vi "XML Read.vi"(8 "error in":errorcluster, 11 "XML File Path In":path) -> (0 "error out":errorcluster, 3 "FOFB Parameters":T1)   [LabVIEW 2011, in "XML VIs.lvlib"]
doc: "Reads an XML file coitaning the FOFB configuration parameters and builds a raw configuration cluster (FOFB Parameters)."
uses:
  XML VIs.lvlib
  Types Definitions/Type FOFB Parameters.ctl
  Types Definitions/Type Network Configuration.ctl
  Types Definitions/Type FA Configuration.ctl
  Types Definitions/Type Response Matrix Measurement Configuration.ctl
  Types Definitions/Type Correction Algorithm Configuration.ctl
  Types Definitions/Type Acquisition Network Configuration.ctl
  Types Definitions/Type Actuation Network Configuration.ctl
  Third Party/GXML/_subVIis/GXML SearchParser/gxml_SearchParser.vi
  Third Party/GXML/GXML.lvlib
  Type Definitions.lvlib
  Controller VIs.lvlib
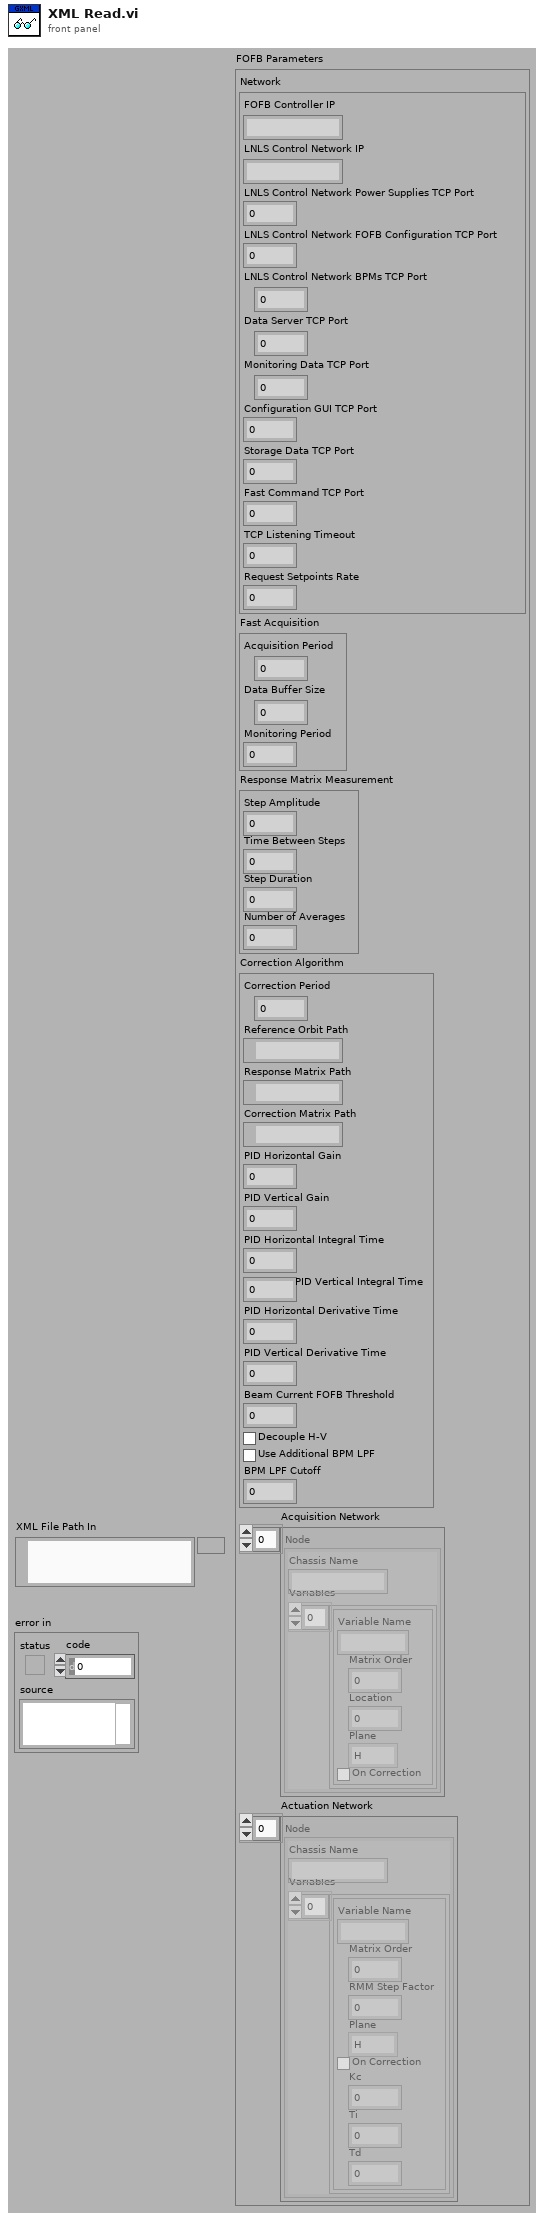
[diagram p1: front panel]
types:
  T1 = typedef "Type Definitions.lvlib/Type FOFB Parameters.ctl" = cluster{"Network":T2, "Fast Acquisition":T3, "Response Matrix Measurement":T4, "Correction Algorithm":T5, "Acquisition Network":T6, "Actuation Network":T7}
  T2 = typedef "Type Definitions.lvlib/Type Network Configuration.ctl" = cluster{"FOFB Controller IP":string, "LNLS Control Network IP":string, "LNLS Control Network Power Supplies TCP Port":u16, "LNLS Control Network FOFB Configuration TCP Port":u16, "LNLS Control Network BPMs TCP Port":u16, "Data Server TCP Port":u16, "Monitoring Data TCP Port":u16, "Configuration GUI TCP Port":u16, "Storage Data TCP Port":u16, "Fast Command TCP Port":u16, "TCP Listening Timeout":i32, "Request Setpoints Rate":u16}
  T3 = typedef "Type Definitions.lvlib/Type FA Configuration.ctl" = cluster{"Acquisition Period":u32, "Data Buffer Size":u32, "Monitoring Period":u32}
  T4 = typedef "Type Definitions.lvlib/Type Response Matrix Measurement Configuration.ctl" = cluster{"Step Amplitude":dbl, "Time Between Steps":u32, "Step Duration":u32, "Number of Averages":u32}
  T5 = typedef "Type Definitions.lvlib/Type Correction Algorithm Configuration.ctl" = cluster{"Correction Period":u32, "Reference Orbit Path":path, "Response Matrix Path":path, "Correction Matrix Path":path, "PID Horizontal Gain":dbl, "PID Vertical Gain":dbl, "PID Horizontal Integral Time":dbl, "PID Vertical Integral Time":dbl, "PID Horizontal Derivative Time":dbl, "PID Vertical Derivative Time":dbl, "Beam Current FOFB Threshold":dbl, "Decouple H-V":bool, "Use Additional BPM LPF":bool, "BPM LPF Cutoff":dbl}
  T6 = typedef "Type Definitions.lvlib/Type Acquisition Network Configuration.ctl" = cluster{"Chassis Name":string, "Variables":cluster{"Variable Name":string, "Matrix Order":u32, "Location":dbl, "Plane":enum8{"H", "V"}, "On Correction":bool}[]}[]
  T7 = typedef "Type Definitions.lvlib/Type Actuation Network Configuration.ctl" = cluster{"Chassis Name":string, "Variables":cluster{"Variable Name":string, "Matrix Order":u32, "RMM Step Factor":dbl, "Plane":enum8{"H", "V"}, "On Correction":bool, "Kc":dbl, "Ti":dbl, "Td":dbl}[]}[]
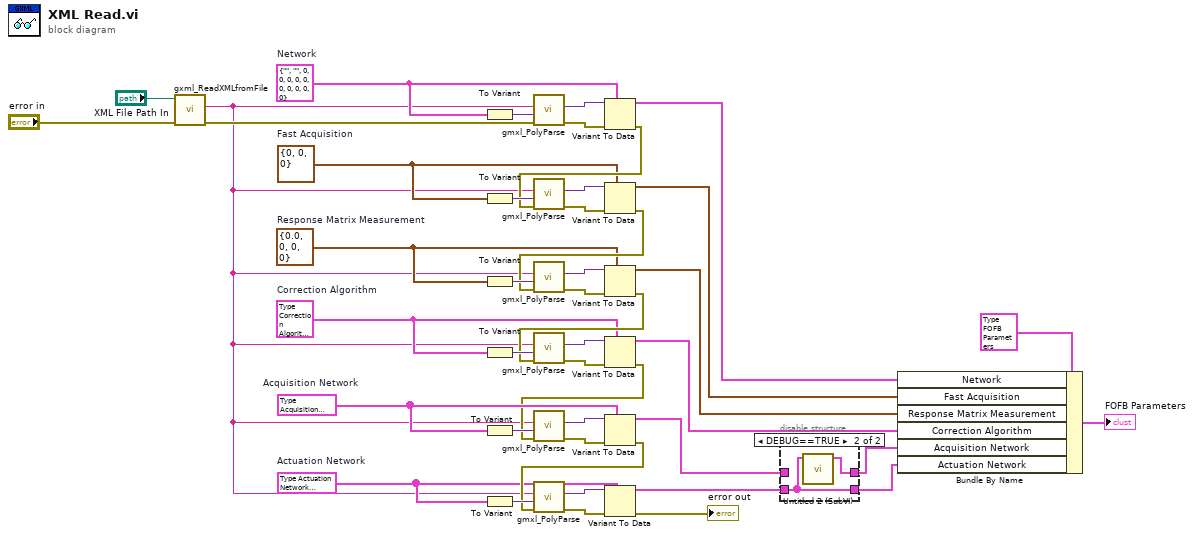
[diagram p0: block diagram]
diagram:
  w6 = T5 {"Correction Period"=0, "Reference Orbit Path"=path "", "Response Matrix Path"=path "", "Correction Matrix Path"=path "", "PID Horizontal Gain"=0.0, "PID Vertical Gain"=0.0, "PID Horizontal Integral Time"=0.0, "PID Vertical Integral Time"=0.0, "PID Horizontal Derivative Time"=0.0, "PID Vertical Derivative Time"=0.0, "Beam Current FOFB Threshold"=0.0, "Decouple H-V"=FALSE, "Use Additional BPM LPF"=FALSE, "BPM LPF Cutoff"=0.0}  # Correction Algorithm
  w12 = T3 {"Acquisition Period"=0, "Data Buffer Size"=0, "Monitoring Period"=0}  # Fast Acquisition
  w13 = T2 {"FOFB Controller IP"="", "LNLS Control Network IP"="", "LNLS Control Network Power Supplies TCP Port"=0, "LNLS Control Network FOFB Configuration TCP Port"=0, "LNLS Control Network BPMs TCP Port"=0, "Data Server TCP Port"=0, "Monitoring Data TCP Port"=0, "Configuration GUI TCP Port"=0, "Storage Data TCP Port"=0, "Fast Command TCP Port"=0, "TCP Listening Timeout"=0, "Request Setpoints Rate"=0}  # Network
  w9 = T4 {"Step Amplitude"=0.0, "Time Between Steps"=0, "Step Duration"=0, "Number of Averages"=0}  # Response Matrix Measurement
  w34 = T7 [{"Chassis Name"="", "Variables"=[{"Variable Name"="", "Matrix Order"=0, "RMM Step Factor"=0.0, "Plane"=enum."H", "On Correction"=FALSE, "Kc"=0.0, "Ti"=0.0, "Td"=0.0}, {"Variable Name"="", "Matrix Order"=0, "RMM Step Factor"=0.0, "Plane"=enum."H", "On Correction"=FALSE, "Kc"=0.0, "Ti"=0.0, "Td"=0.0}, {"Variable Name"="", "Matrix Order"=0, "RMM Step Factor"=0.0, "Plane"=enum."H", "On Correction"=FALSE, "Kc"=0.0, "Ti"=0.0, "Td"=0.0}, {"Variable Name"="", "Matrix Order"=0, "RMM Step Factor"=0.0, "Plane"=enum."H", "On Correction"=FALSE, "Kc"=0.0, "Ti"=0.0, "Td"=0.0}, {"Variable Name"="", "Matrix Order"=0, "RMM Step Factor"=0.0, "Plane"=enum."H", "On Correction"=FALSE, "Kc"=0.0, "Ti"=0.0, "Td"=0.0}, {"Variable Name"="", "Matrix Order"=0, "RMM Step Factor"=0.0, "Plane"=enum."H", "On Correction"=FALSE, "Kc"=0.0, "Ti"=0.0, "Td"=0.0}, {"Variable Name"="", "Matrix Order"=0, "RMM Step Factor"=0.0, "Plane"=enum."H", "On Correction"=FALSE, "Kc"=0.0, "Ti"=0.0, "Td"=0.0}, {"Variable Name"="", "Matrix Order"=0, "RMM Step Factor"=0.0, "Plane"=enum."H", "On Correction"=FALSE, "Kc"=0.0, "Ti"=0.0, "Td"=0.0}]}]  # Actuation Network
  w35 = T6 [{"Chassis Name"="", "Variables"=[{"Variable Name"="", "Matrix Order"=0, "Location"=0.0, "Plane"=enum."H", "On Correction"=FALSE}, {"Variable Name"="", "Matrix Order"=0, "Location"=0.0, "Plane"=enum."H", "On Correction"=FALSE}, {"Variable Name"="", "Matrix Order"=0, "Location"=0.0, "Plane"=enum."H", "On Correction"=FALSE}, {"Variable Name"="", "Matrix Order"=0, "Location"=0.0, "Plane"=enum."H", "On Correction"=FALSE}, {"Variable Name"="", "Matrix Order"=0, "Location"=0.0, "Plane"=enum."H", "On Correction"=FALSE}, {"Variable Name"="", "Matrix Order"=0, "Location"=0.0, "Plane"=enum."H", "On Correction"=FALSE}, {"Variable Name"="", "Matrix Order"=0, "Location"=0.0, "Plane"=enum."H", "On Correction"=FALSE}, {"Variable Name"="", "Matrix Order"=0, "Location"=0.0, "Plane"=enum."H", "On Correction"=FALSE}]}]  # Acquisition Network
  n1 = call "gxml_ReadXMLfromFile.vi"("error in"="error in", "XML File Path"="XML File Path In") -> ("error out"=w19:errorcluster, "XML String Out"=w5:string)  [unwired: 7 in, 1 out]
  n2 = To Variant(anything=w13) -> (Variant=w20:variant)
  n3 = To Variant(anything=w12) -> (Variant=w25:variant)
  n4 = To Variant(anything=w9) -> (Variant=w31:variant)
  n5 = To Variant(anything=w6) -> (Variant=w30:variant)
  n6 = To Variant(anything=w35) -> (Variant=w43:variant)
  n7 = To Variant(anything=w34) -> (Variant=w38:variant)
  n8 = call-poly "gmxl_PolyParse.vi"("error in"=w19, "TypeDesc"=w20, "XML String In"=w5) -> ("error out"=w22:errorcluster, "Parsed Data"=w21:variant)  [unwired: 7 in]
  n9 = Variant To Data(error in=w22, type=w13, Variant=w21) -> (data=w10:T2, error out=w18:errorcluster)
  n10 = call-poly "gmxl_PolyParse.vi"("error in"=w18, "TypeDesc"=w25, "XML String In"=w5) -> ("error out"=w23:errorcluster, "Parsed Data"=w24:variant)  [unwired: 7 in]
  n11 = Variant To Data(error in=w23, type=w12, Variant=w24) -> (data=w11:T3, error out=w14:errorcluster)
  n12 = call-poly "gmxl_PolyParse.vi"("error in"=w14, "TypeDesc"=w31, "XML String In"=w5) -> ("error out"=w33:errorcluster, "Parsed Data"=w32:variant)  [unwired: 7 in]
  n13 = Variant To Data(error in=w33, type=w9, Variant=w32) -> (data=w7:T4, error out=w27:errorcluster)
  n14 = call-poly "gmxl_PolyParse.vi"("error in"=w27, "TypeDesc"=w30, "XML String In"=w5) -> ("error out"=w28:errorcluster, "Parsed Data"=w29:variant)  [unwired: 7 in]
  n15 = Variant To Data(error in=w28, type=w6, Variant=w29) -> (data=w8:T5, error out=w26:errorcluster)
  n16 = call-poly "gmxl_PolyParse.vi"("error in"=w26, "TypeDesc"=w43, "XML String In"=w5) -> ("error out"=w41:errorcluster, "Parsed Data"=w42:variant)  [unwired: 7 in]
  n17 = Variant To Data(error in=w41, type=w35, Variant=w42) -> (data=w2:T6, error out=w37:errorcluster)
  n18 = call-poly "gmxl_PolyParse.vi"("error in"=w37, "TypeDesc"=w38, "XML String In"=w5) -> ("error out"=w40:errorcluster, "Parsed Data"=w39:variant)  [unwired: 7 in]
  n19 = Variant To Data(error in=w40, type=w34, Variant=w39) -> (data=w4:T7, error out=→"error out":errorcluster)
  n20 = disable-structure shown="DEBUG==TRUE" {
    disable-tunnel: w4 -> [w46 w47]
    disable-tunnel: [w46 w47] -> w3
    disable-tunnel: [w45 w48] -> w1
    disable-tunnel: w2 -> [w45 _]
    frame condition #0 {
    }
    frame condition #1 (active) {
      n21 = call "Untitled 2 (SubVI).vi"("Actuation Network"=w47) -> ("Acquisition Network"=w48:T6)  [unwired: 10 in]
    }
  }
  n22 = Bundle By Name(cluster=T1 {"Network"={"FOFB Controller IP"="", "LNLS Control Network IP"="", "LNLS Control Network Power Supplies TCP Port"=0, "LNLS Control Network FOFB Configuration TCP Port"=0, "LNLS Control Network BPMs TCP Port"=0, "Data Server TCP Port"=0, "Monitoring Data TCP Port"=0, "Configuration GUI TCP Port"=0, "Storage Data TCP Port"=0, "Fast Command TCP Port"=0, "TCP Listening Timeout"=0, "Request Setpoints Rate"=0}, "Fast Acquisition"={"Acquisition Period"=0, "Data Buffer Size"=0, "Monitoring Period"=0}, "Response Matrix Measurement"={"Step Amplitude"=0.0, "Time Between Steps"=0, "Step Duration"=0, "Number of Averages"=0}, "Correction Algorithm"={"Correction Period"=0, "Reference Orbit Path"=path "", "Response Matrix Path"=path "", "Correction Matrix Path"=path "", "PID Horizontal Gain"=0.0, "PID Vertical Gain"=0.0, "PID Horizontal Integral Time"=0.0, "PID Vertical Integral Time"=0.0, "PID Horizontal Derivative Time"=0.0, "PID Vertical Derivative Time"=0.0, "Beam Current FOFB Threshold"=0.0, "Decouple H-V"=FALSE, "Use Additional BPM LPF"=FALSE, "BPM LPF Cutoff"=0.0}, "Acquisition Network"=[], "Actuation Network"=[]} ("FOFB Parameters"), "Network"=w10, "Fast Acquisition"=w11, "Response Matrix Measurement"=w7, "Correction Algorithm"=w8, "Acquisition Network"=w1, "Actuation Network"=w3) -> (→"FOFB Parameters":T1)
